vi "velodynepaser.vi"(0 "roll":dbl=0.5000000000000001, 1 "pitch":dbl=-6.0, 2 "heading":dbl=1.2, 3 "dX":dbl=-0.009999999999999997, 4 "dY":dbl=1.287, 5 "dZ":dbl=1.6) -> (14 "size":i32, 17 "pos_velo":dbl[](array[numeric]))   [LabVIEW 2015]
uses:
  G_SEN.vi
  <vilib>/Analysis/Matrix/Numeric/Conversions/Array To Matrix - RA2.vi
  <vilib>/Analysis/Matrix/Numeric/Multiply/Multiply - RM,RM.vi
  <vilib>/Analysis/Matrix/NI_Matrix.lvlib
panel:
  out "d":dbl[](array[numeric])
  out "i":u8[](array[numeric])
  out "y":dbl[](array[numeric])
  out "x":dbl[](array[numeric])
  out "z":dbl[](array[numeric])
  in  "thresh":dbl
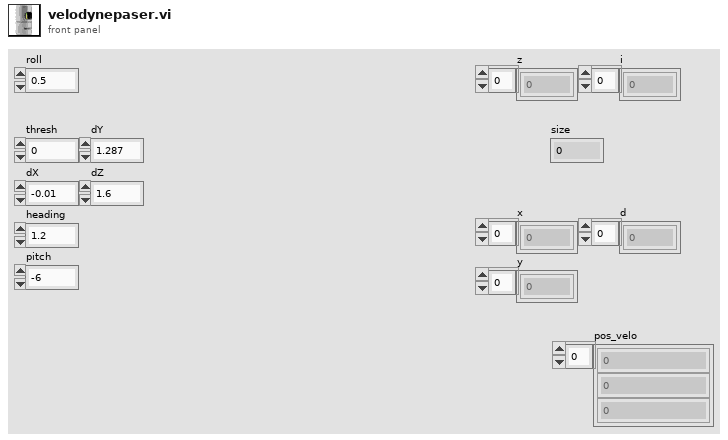
[diagram p1: front panel]
types:
  T1 = typedef "NI_Matrix.lvlib/RealMatrix.ctl" = dbl[][]
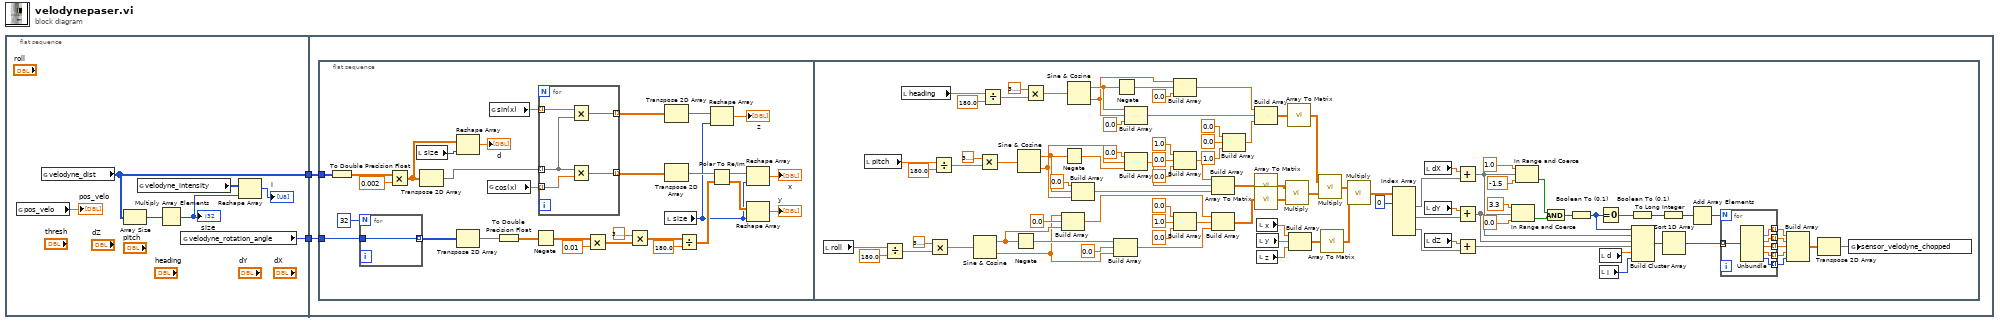
[diagram p0: block diagram]
diagram:
  n1 = flat-sequence {
    tunnel: [w9] -> w2
    tunnel: [w8] -> w1
    tunnel: w2 -> [w11]
    tunnel: w1 -> [w10]
    frame #0 {
      n2 = global read "G_SEN.vi" "pos_velo"() -> (→"pos_velo":dbl[])
      n3 = global read "G_SEN.vi" "velodyne_dist"() -> (w8:u16[][])
      n4 = Array Size(array=w8) -> (size(s)=w7:i32[])
      n5 = global read "G_SEN.vi" "velodyne_intensity"() -> (w5:u8[][])
      n6 = Multiply Array Elements(1:w7) -> (0:w4:i32)
      "size" <- w4
      n7 = global read "G_SEN.vi" "velodyne_rotation_angle"() -> (w9:u16[])
      n8 = Reshape Array(w5, w4) -> (→"i":u8[])
    }
    frame #1 {
      n9 = flat-sequence {
        tunnel: w11 -> [w38]
        tunnel: w10 -> [w23]
        frame #0 {
          n10 = To Double Precision Float(number=w23) -> (double precision float=w25:dbl[][])
          n11 = for {
            N: 32 -> [_]
            tunnel: w38 -> [w48]
            tunnel: [w48] -> w36 mode=indexing
          }
          n12 = Multiply(x=w25, y=0.002) -> (x*y=w24:dbl[][])
          n13 = local read "size"() -> (w22:i32)
          n14 = Transpose 2D Array(2D array=w24) -> (transposed array=w33:dbl[][])
          n15 = Reshape Array(w24, w22) -> (→"d":dbl[])
          n16 = Transpose 2D Array(2D array=w36) -> (transposed array=w35:u16[][])
          n17 = global read "G_SEN.vi" "cos(x)"() -> (w32:dbl[])
          n18 = global read "G_SEN.vi" "sin(x)"() -> (w18:dbl[])
          n19 = To Double Precision Float(number=w35) -> (double precision float=w20:dbl[][])
          n20 = Negate(x=w20) -> (-x=w12:dbl[][])
          n21 = for {
            tunnel: w33 -> [w44] mode=indexing
            tunnel: w32 -> [w47] mode=indexing
            tunnel: [w46] -> w31 mode=indexing
            tunnel: w18 -> [w45] mode=indexing
            tunnel: [w43] -> w28 mode=indexing
            n22 = Multiply(x=w45, y=w44) -> (x*y=w43:dbl[])
            n23 = Multiply(x=w44, y=w47) -> (x*y=w46:dbl[])
          }
          n24 = Multiply(x=w12, y=0.01) -> (x*y=w19:dbl[][])
          n25 = Multiply(x=3.141592653589793, y=w19) -> (x*y=w40:dbl[][])
          n26 = Transpose 2D Array(2D array=w28) -> (transposed array=w27:dbl[][])
          n27 = Transpose 2D Array(2D array=w31) -> (transposed array=w29:dbl[][])
          n28 = local read "size"() -> (w13:i32)
          n29 = Divide(x=w40, y=180.0) -> (x/y=w34:dbl[][])
          n30 = Reshape Array(w27, w13) -> (→"z":dbl[])
          n31 = Polar To Re/Im(2:w34, 3:w29) -> (0:w21:dbl[][], 1:w26:dbl[][])
          n32 = Reshape Array(w26, w13) -> (→"x":dbl[])
          n33 = Reshape Array(w21, w13) -> (→"y":dbl[])
        }
        frame #1 {
          n34 = local read "roll"() -> (w76:dbl)
          n35 = local read "pitch"() -> (w85:dbl)
          n36 = Divide(x=w76, y=180.0) -> (x/y=w78:dbl)
          n37 = local read "heading"() -> (w80:dbl)
          n38 = Multiply(x=3.141592653589793, y=w78) -> (x*y=w74:dbl)
          n39 = Divide(x=w85, y=180.0) -> (x/y=w88:dbl)
          n40 = Sine & Cosine(0:w74) -> (1:w130:dbl, 2:w127:dbl)
          n41 = Multiply(x=3.141592653589793, y=w88) -> (x*y=w84:dbl)
          n42 = Divide(x=w80, y=180.0) -> (x/y=w81:dbl)
          n43 = Negate(x=w130) -> (-x=w129:dbl)
          n44 = Sine & Cosine(0:w84) -> (1:w114:dbl, 2:w117:dbl)
          n45 = Multiply(x=3.141592653589793, y=w81) -> (x*y=w79:dbl)
          n46 = Build Array(w127, 0.0 ("element"), w130) -> (w132:dbl[])
          n47 = Negate(x=w114) -> (-x=w116:dbl)
          n48 = Sine & Cosine(0:w79) -> (1:w111:dbl, 2:w109:dbl)
          n49 = Build Array(0.0 ("element"), w114, w117) -> (w113:dbl[])
          n50 = Build Array(w129, 0.0 ("element"), w127) -> (w126:dbl[])
          n51 = Negate(x=w111) -> (-x=w110:dbl)
          n52 = Build Array(w111, w109, 0.0 ("element")) -> (w112:dbl[])
          n53 = Build Array(0.0 ("element"), w117, w116) -> (w119:dbl[])
          n54 = Build Array(w109, w110, 0.0 ("element")) -> (w108:dbl[])
          n55 = Build Array(1.0 ("element"), 0.0 ("element"), 0.0 ("element")) -> (w120:dbl[])
          n56 = Build Array(0.0 ("element"), 1.0 ("element"), 0.0 ("element")) -> (w131:dbl[])
          n57 = Build Array(w120, w119, w113) -> (w124:dbl[][])
          n58 = Build Array(w132, w131, w126) -> (w125:dbl[][])
          n59 = Build Array(0.0 ("element"), 0.0 ("element"), 1.0 ("element")) -> (w103:dbl[])
          n60 = Build Array(w108, w112, w103) -> (w104:dbl[][])
          n61 = call-poly <vilib>:"Array To Matrix.vi"("Real 2D Array"=w124) -> ("Real Matrix"=w99:T1)
          n62 = call-poly <vilib>:"Array To Matrix.vi"("Real 2D Array"=w125) -> ("Real Matrix"=w100:T1)
          n63 = local read "x"() -> (w96:dbl[])
          n64 = local read "y"() -> (w95:dbl[])
          n65 = local read "z"() -> (w94:dbl[])
          n66 = call-poly <vilib>:"Multiply.vi"("Real Matrix B"=w100, "Real Matrix A"=w99) -> ("A * B"=w98:T1)
          n67 = call-poly <vilib>:"Array To Matrix.vi"("Real 2D Array"=w104) -> ("Real Matrix"=w97:T1)
          n68 = Build Array(w96, w95, w94) -> (w93:dbl[][])
          n69 = call-poly <vilib>:"Multiply.vi"("Real Matrix B"=w98, "Real Matrix A"=w97) -> ("A * B"=w92:T1)
          n70 = call-poly <vilib>:"Array To Matrix.vi"("Real 2D Array"=w93) -> ("Real Matrix"=w91:T1)
          n71 = call-poly <vilib>:"Multiply.vi"("Real Matrix B"=w91, "Real Matrix A"=w92) -> ("A * B"=w90:T1)
          n72 = Index Array(array=w90, index (row) #1=0 ("index (row)")) -> (element #1=w139:dbl[], element #2=w141:dbl[], element #3=w143:dbl[])  [unwired: 5 in]
          n73 = local read "dX"() -> (w138:dbl)
          n74 = local read "dY"() -> (w140:dbl)
          n75 = local read "dZ"() -> (w142:dbl)
          n76 = Add(x=w138, y=w139) -> (x+y=w65:dbl[])
          n77 = Add(x=w140, y=w141) -> (x+y=w56:dbl[])
          n78 = Add(x=w142, y=w143) -> (x+y=w137:dbl[])
          n79 = In Range and Coerce(upper limit=3.3, x=w56, lower limit=0.0) -> (In Range?=w67:bool[])  [unwired: 1 out]
          n80 = In Range and Coerce(upper limit=1.0, x=w65, lower limit=-1.5) -> (In Range?=w70:bool[])  [unwired: 1 out]
          n81 = And(x=w70, y=w67) -> (x .and. y?=w66:bool[])
          n82 = Boolean To (0,1)(Boolean=w66) -> (0, 1=w61:i16[])
          n83 = Equal To 0?(x=w61) -> (x = 0?=w60:bool[])
          n84 = local read "d"() -> (w64:dbl[])
          n85 = local read "i"() -> (w63:u8[])
          n86 = Boolean To (0,1)(Boolean=w60) -> (0, 1=w50:i16[])
          n87 = Build Cluster Array(w61, w65, w56, w137, w64, w63) -> (w62:cluster{i16, dbl, dbl, dbl, dbl, "element":u8}[])
          n88 = To Long Integer(number=w50) -> (32bit integer=w49:i32[])
          n89 = Sort 1D Array(array=w62) -> (sorted array=w58:cluster{i16, dbl, dbl, dbl, dbl, "element":u8}[])
          n90 = Add Array Elements(numeric array=w49) -> (sum=w59:i32)
          n91 = for {
            N: w59 -> [_]
            tunnel: w58 -> [w149] mode=indexing
            tunnel: [w148] -> w57 mode=indexing
            tunnel: [w147] -> w55 mode=indexing
            tunnel: [w146] -> w54 mode=indexing
            tunnel: [w145] -> w53 mode=indexing
            tunnel: [w144] -> w52 mode=indexing
            n92 = Unbundle(w149) -> (w148:dbl, w147:dbl, w146:dbl, w145:dbl, "element"=w144:u8)  [unwired: 1 out]
          }
          n93 = Build Array(w57, w55, w54, w53, w52) -> (w73:dbl[][])
          n94 = Transpose 2D Array(2D array=w73) -> (transposed array=w51:dbl[][])
          n95 = global write "G_SEN.vi" "sensor_velodyne_chopped"(w51) -> ()
        }
      }
    }
  }
